vi "DN-Start.vi"   [LabVIEW 2015]
uses:
  Packages/CSPP_Core/Actors/CS++StartActor/CS++StartActor.lvlib
types:
  T1 = cluster{"Classname":string, "CS++Messages":refnum<class "Message.lvclass">[]}[]
  T2 = enum32{"invalid app kind", "Development System", "Run Time System", "Student Edition", "Embedded LabVIEW", "Evaluation", "Custom"}
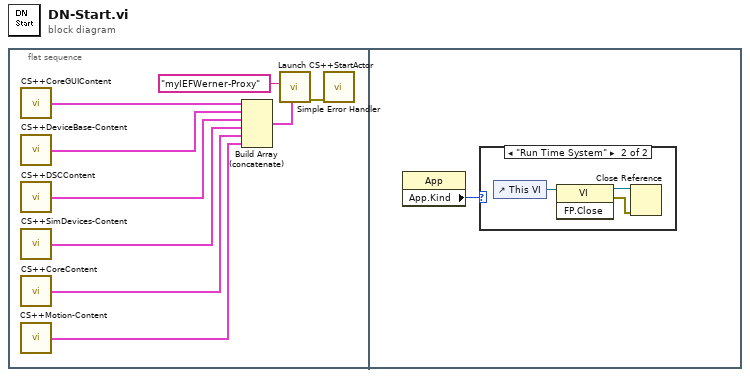
[diagram p0: block diagram]
diagram:
  n1 = flat-sequence {
    frame #0 {
      n2 = call "CS++CoreGUIContent.vi"() -> ("CS++Classes & Messages"=w8:T1)  [unwired: 1 in]
      n3 = call "CS++DeviceBase-Content.vi"() -> ("CS++Classes & Messages"=w7:T1)  [unwired: 1 in]
      n4 = call "CS++DSCContent.vi"() -> ("CS++Classes & Messages"=w6:T1)  [unwired: 1 in]
      n5 = call "CS++SimDevices-Content.vi"() -> ("CS++Classes & Messages"=w5:T1)  [unwired: 1 in]
      n6 = call "CS++CoreContent.vi"() -> ("CS++Classes & Messages"=w3:T1)  [unwired: 1 in]
      n7 = call "CS++Motion-Content.vi"() -> ("CS++Classes & Messages"=w2:T1)  [unwired: 1 in]
      n8 = Build Array (concatenate)(w8, w7, w6, w5, w3, w2) -> (w9:T1)
      n9 = call "Launch CS++StartActor.vi"("CS++Classes & Messages"=w9, "Start Actor"="myIEFWerner-Proxy") -> ("Error Out"=w1:errorcluster)  [unwired: 7 in, 2 out]
      n10 = call <vilib>:"Simple Error Handler.vi"("error in (no error)"=w1) -> ()  [unwired: 4 in, 5 out]
    }
    frame #1 {
      n11 = property class="App"() -> ("App.Kind"=w10:T2)  [unwired: 2 in, 2 out]
      n12 = case shown="\"Run Time System\"" w10 {
        frame Default {
        }
        frame "Run Time System" {
          n13 = control-ref of="This VI"() -> (w13:refnum<vi>)
          n14 = invoke class="VI" method="FP.Close"(reference=w13) -> (reference out=w12:refnum<vi>, error out=w11:errorcluster)  [unwired: 2 in, 1 out]
          n15 = Close Reference(reference=w12, error in (no error)=w11) -> ()  [unwired: 1 out]
        }
      }
    }
  }
